vi "sine demod.vi"() -> ()   [LabVIEW 2014]
panel:
  out "Init Data Out":fxp<+/-,2,2>[](array[numeric])=[1.0, 0.0, -1.0, 0.0]
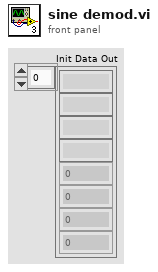
[diagram p1: front panel]
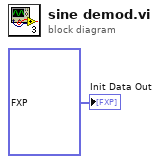
[diagram p0: block diagram]
diagram:
  "Init Data Out" <- fxp<+/-,2,2>[] [0.0, -1.0, 0.0, 1.0] ("Init Data Out")
